vi "snap_usrp_rx.vi"() -> ()   [LabVIEW 2014]
uses:
  <vilib>/vision/Image Controls.llb/IMAQ Image.ctl
  <vilib>/addons/Modulation/Analog/support/mod_Set Error Source.vi
  var_rx_stop.vi
  <vilib>/addons/Modulation/Digital/Support/Common/Validators/mod_Generate Filter Coefficients Validate.vi
  <vilib>/addons/Modulation/Digital/General/subVIs/mod_Generate Filter Coefficients.vi
  <instrlib>/niUSRP/niUSRP Fetch Rx Data (CDB Cluster).vi
  <vilib>/addons/Modulation/niDMT.lvlib
panel:
  out "total_pkts":u32
  in  "arity":enum16{"binary", "quadrature"}(ring)
  out "Image":T1(plugin-control)
  out "# elements in queue":i32
  in  "queue limit":i32
  out "error IO":errorcluster
  in  "number of samples":i64=100000
  in  "Clocking and Synchronization:Timebase Clock Source":string(combo)="Internal"
  in  "Clocking and Synchronization:Reference Frequency Source":string(combo)="Internal"
  in  "Active Channel":string
  in  "active antenna":string
  in  "gain":dbl format="%#_6f"
  in  "carrier frequency":dbl=100000.0 format="%#_6p"
  in  "IQ rate":dbl=100000.0 format="%#_6p"
  in  "device names":refnum<k15>
  in  "stop":bool
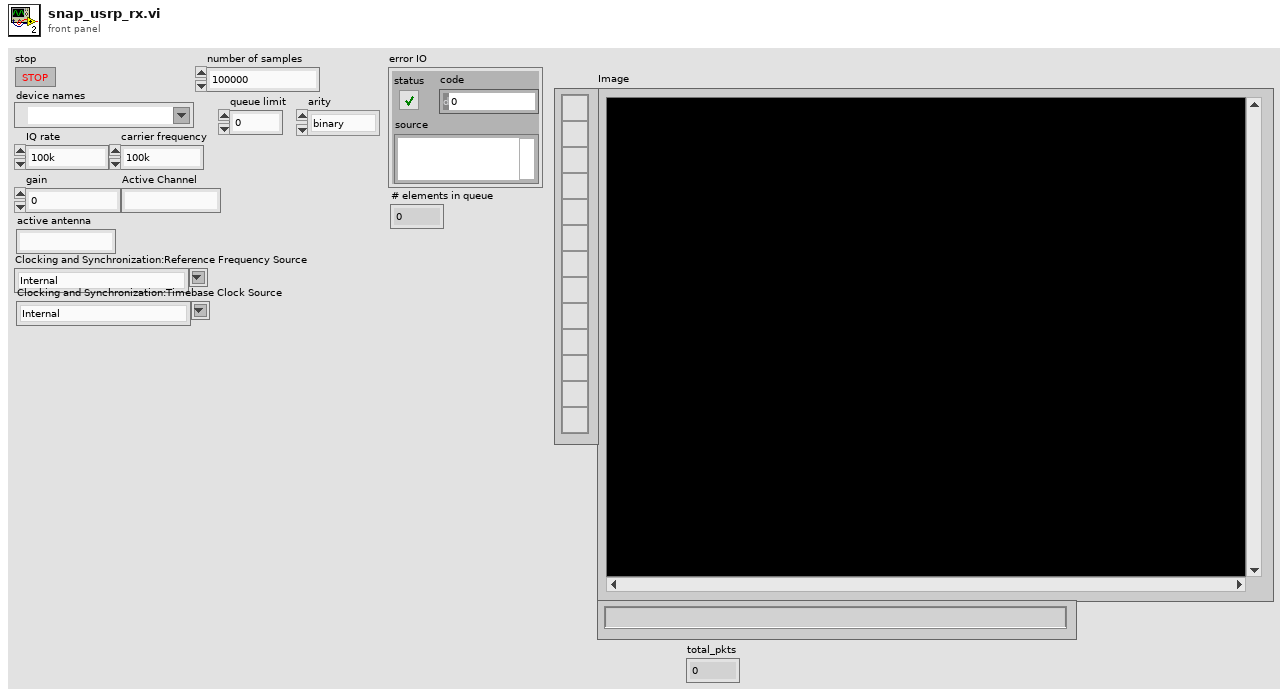
[diagram p1: front panel]
types:
  T1 = typedef "IMAQ Image.ctl" = refnum<image>
  T2 = enum16{"none", "Raised Cosine", "Root Raised Cos", "Gaussian"}
  T3 = enum16{"FSK", "PSK", "QAM", "MSK", "PAM", "ASK", "CPM"}
  T4 = cluster{"pkt_idx":u32, "pkt_size":u32, "payload":string}[]
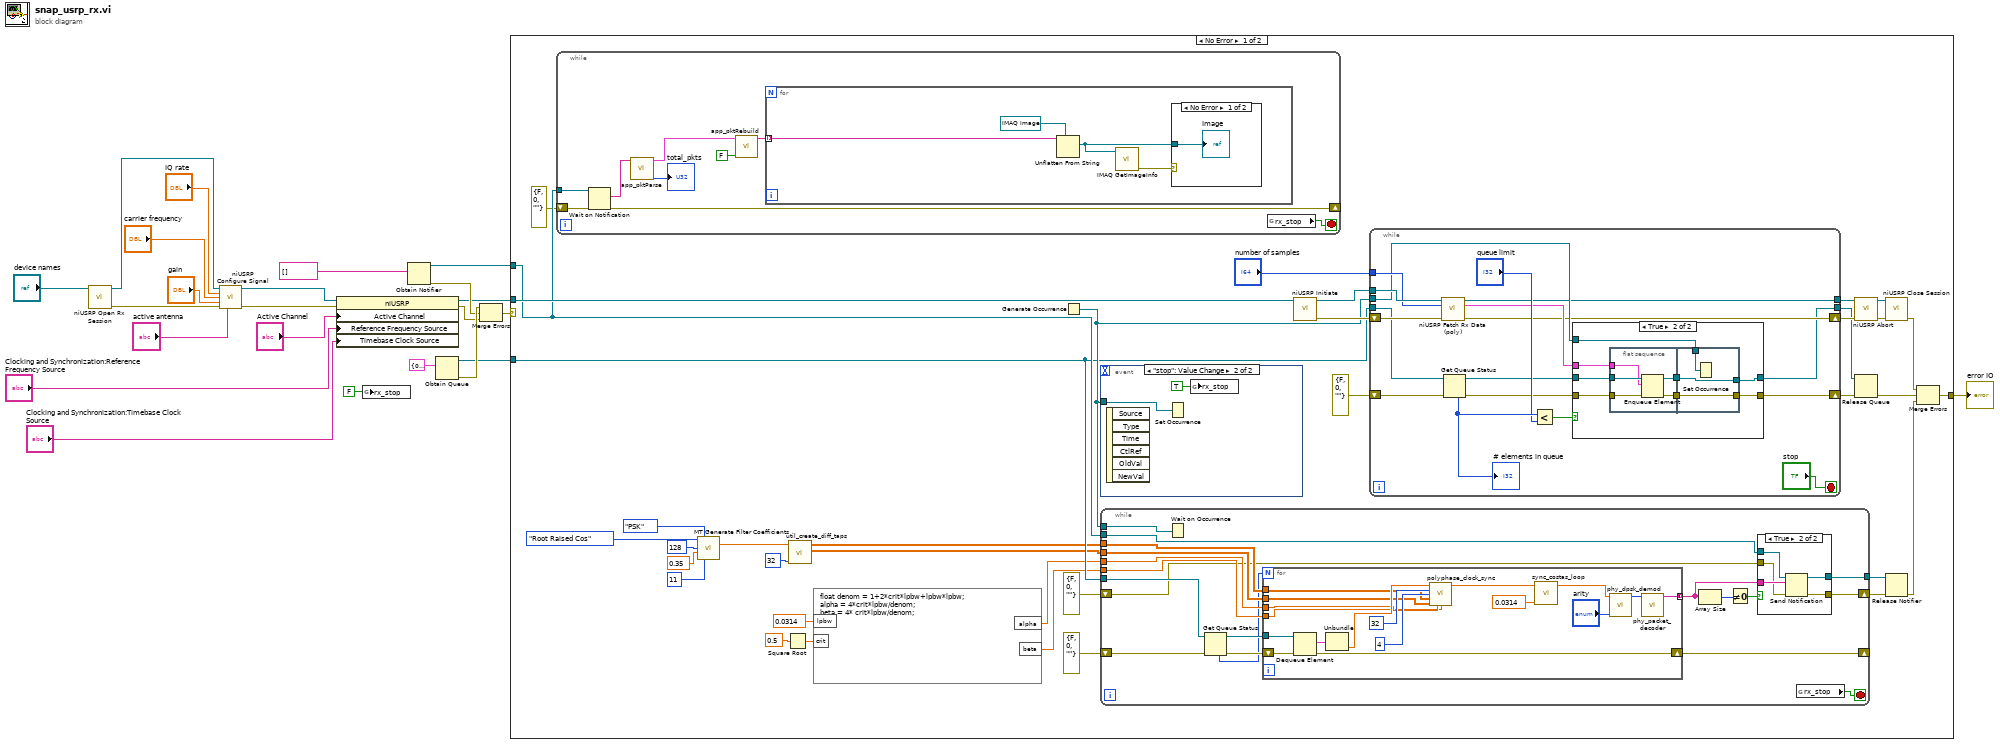
[diagram p0: block diagram]
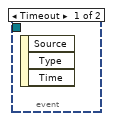
[diagram p5: hidden frame]
diagram:
  n1 = call <instrlib>:"niUSRP Open Rx Session.vi"("device names"="device names") -> ("session handle out"=w22:refnum<k15>, "error out"=w21:errorcluster)  [unwired: 13 in]
  n2 = call <instrlib>:"niUSRP Configure Signal.vi"("session handle"=w22, "IQ rate"="IQ rate", "carrier frequency"="carrier frequency", "gain"="gain", "error in (no error)"=w21, "active antenna"="active antenna") -> ("session handle out"=w20:refnum<k15>, "error out"=w19:errorcluster)  [unwired: 5 in, 3 out]
  n3 = property class="niUSRP"(reference=w20, error in=w19, "Active Channel"="Active Channel", "Reference Frequency Source"="Clocking and Synchronization:Reference Frequency Source", "Timebase Clock Source"="Clocking and Synchronization:Timebase Clock Source") -> (reference out=w6:refnum<k15>, error out=w16:errorcluster)
  n4 = global write "var_rx_stop.vi" "rx_stop"(FALSE) -> ()
  n5 = Obtain Notifier(notification data type=string[] []) -> (notifier out=w3:refnum<notifier>, error out=w17:errorcluster)  [unwired: 3 in, 1 out]
  n6 = Obtain Queue(element data type=cluster{"t0":dbl, "dt":dbl, "Y":cdb[]} {"t0"=0.0, "dt"=0.0, "Y"=[]} ("data")) -> (queue out=w4:refnum<queue>, error out=w18:errorcluster)  [unwired: 4 in, 1 out]
  n7 = Merge Errors(w18, w17, w16) -> (w15:errorcluster)
  n8 = case shown="No Error" w15 {
    selector: w15 -> [_ w155]
    tunnel: w6 -> [w60 _]
    tunnel: w4 -> [w38 _]
    tunnel: w3 -> [w47 _]
    tunnel: [w42 w155] -> w2
    frame No Error {
      n9 = while {
        tunnel: w47 -> [w68]
        shift-right: [w66] -> _
        shift-left: errorcluster {"status"=FALSE, "code"=0, "source"=""} ("error out") -> [w67]
        stop <- w69 stop-if-true
        n10 = Wait on Notification(notifier=w68, error in (no error)=w67) -> (notification=w65:string[], error out=w66:errorcluster)  [unwired: 2 in, 2 out]
        n11 = call "app_pktParse.vi"("pkts_get"=w65) -> ("total_pkts"=→"total_pkts":u32, "app_pkt"=w64:T4)  [unwired: 9 in]
        n12 = call "app_pktRebuild.vi"("reset"=FALSE, "app_pkt"=w64) -> ("out pkts"=w61:string[])  [unwired: 9 in]
        n13 = for {
          tunnel: w61 -> [w73] mode=indexing
          n14 = Unflatten From String(type=T1 refnum ("Image"), binary string=w73) -> (value=w70:T1)  [unwired: 3 in, 2 out]
          n15 = call "IMAQ GetImageInfo"("Image"=w70) -> ("error out"=w71:errorcluster)  [unwired: 3 in, 7 out]
          n16 = case shown="No Error" w71 {
            tunnel: w70 -> [w74 _]
            frame No Error {
              "Image" <- w74
            }
            frame Error {
            }
          }
        }
        n17 = global read "var_rx_stop.vi" "rx_stop"() -> (w69:bool)
      }
      n18 = call <vilib>:"MT Generate Filter Coefficients.vi"("pulse shaping filter (none)"=T2."Root Raised Cos", "modulation type"=T3."PSK", "matched samples per symbol (16)"=128, "filter parameter"=0.35, "filter length (symbols)"=11) -> ("matched filter coefficients"=w33:dbl[])  [unwired: 8 in, 2 out]
      n19 = Square Root(x=0.5) -> (sqrt(x)=w36:dbl)
      n20 = call "util_create_diff_taps.vi"("nfilts"=32, "taps"=w33) -> ("out diff taps"=w24:dbl[][], "out taps"=w25:dbl[][])  [unwired: 7 in, 1 out]
      n21 = formula code="float denom = 1+2*crit*lpbw+lpbw*lpbw;\nalpha = 4*crit*lpbw/denom;\nbeta = 4* crit*lpbw/denom;"("lpbw"=0.0314 ("input variable"), "crit"=w36) -> ("alpha"=w27:dbl, "beta"=w26:dbl)
      n22 = Generate Occurrence() -> (w56:refnum<k4>)
      n23 = event shown="[1] \"stop\": Value Change" {
        selector: _ -> [_ _]
        dyn-events: _ -> [_ _]
        timeout: _ -> [_ _]
        tunnel: w56 -> [_ w153]
        event Timeout {
          n24 = event-data() -> ()  [unwired: 1 in, 3 out]
        }
        event "stop": Value Change {
          n25 = event-data() -> ()  [unwired: 1 in, 6 out]
          n26 = Set Occurrence(w153) -> ()
          n27 = global write "var_rx_stop.vi" "rx_stop"(TRUE) -> ()
        }
      }
      n28 = while {
        tunnel: w56 -> [w93]
        tunnel: w47 -> [w79]
        tunnel: [w76] -> w52
        shift-right: [w77] -> w51
        shift-left: errorcluster {"status"=FALSE, "code"=0, "source"=""} ("error out") -> [w78]
        shift-right: [w83] -> _
        shift-left: errorcluster {"status"=FALSE, "code"=0, "source"=""} ("error out") -> [w91]
        tunnel: w38 -> [w90]
        tunnel: w25 -> [w87]
        tunnel: w24 -> [w86]
        tunnel: w27 -> [w85]
        tunnel: w26 -> [w84]
        stop <- w92 stop-if-true
        n29 = Wait on Occurrence(2:w93) -> ()  [unwired: 2 in, 1 out]
        n30 = Get Queue Status(queue=w90, error in (no error)=w91) -> (queue out=w89:refnum<queue>, error out=w88:errorcluster, # elements in queue=w75:i32)  [unwired: 1 in, 5 out]
        n31 = for {
          N: w75 -> [_]
          tunnel: w89 -> [w117]
          shift-right: [w101] -> w83
          shift-left: w88 -> [w116]
          tunnel: w87 -> [w109]
          tunnel: w86 -> [w108]
          tunnel: w85 -> [w107]
          tunnel: w84 -> [w106]
          tunnel: [w102] -> w82 mode=concatenating
          n32 = Dequeue Element(queue=w117, error in (no error)=w116) -> (element=w115:cluster{"t0":dbl, "dt":dbl, "Y":cdb[]}, error out=w101:errorcluster)  [unwired: 1 in, 2 out]
          n33 = Unbundle(w115) -> ("Y"=w114:cdb[])  [unwired: 2 out]
          n34 = call "polyphase_clock_sync.vi"("samples"=w114, "nfilts"=32, "sps"=4, "taps"=w109, "diff taps"=w108, "alpha"=w107, "beta"=w106) -> ("out symbols"=w113:cdb[])  [unwired: 7 in, 1 out]
          n35 = call "sync_costas_loop.vi"("loop bandwidth"=0.0314, "symbols"=w113) -> ("outputs"=w112:cdb[])  [unwired: 9 in]
          n36 = call "phy_dpsk_demod.vi"("arity"="arity", "dpsk"=w112) -> ("bitstream"=w103:u8[])  [unwired: 9 in]
          n37 = call "phy_packet_decoder.vi"("bits"=w103) -> ("string Array"=w102:string[])  [unwired: 10 in]
        }
        n38 = Array Size(array=w82) -> (size(s)=w81:i32)
        n39 = Not Equal To 0?(x=w81) -> (x != 0?=w80:bool)
        n40 = case shown="True" w80 {
          tunnel: w82 -> [_ w100]
          tunnel: w79 -> [w95 w99]
          tunnel: w78 -> [w94 w98]
          tunnel: [w94 w97] -> w77
          tunnel: [w95 w96] -> w76
          frame False {
          }
          frame True {
            n41 = Send Notification(notification=w100, notifier=w99, error in (no error)=w98) -> (notifier out=w96:refnum<notifier>, error out=w97:errorcluster)
          }
        }
        n42 = global read "var_rx_stop.vi" "rx_stop"() -> (w92:bool)
      }
      n43 = call <instrlib>:"niUSRP Initiate.vi"("session handle"=w60) -> ("session handle out"=w59:refnum<k15>, "error out"=w58:errorcluster)  [unwired: 13 in]
      n44 = while {
        tunnel: w59 -> [w133]
        tunnel: "number of samples" -> [w131]
        tunnel: w56 -> [w130]
        tunnel: w38 -> [w129]
        shift-right: [w121] -> w53
        shift-left: w58 -> [w132]
        shift-right: [w119] -> w40
        shift-left: errorcluster {"status"=FALSE, "code"=0, "source"=""} ("error out") -> [w128]
        tunnel: [w122] -> w41
        tunnel: [w118] -> w39
        stop <- "stop" stop-if-true
        n45 = call-poly <instrlib>:"niUSRP Fetch Rx Data (poly).vi"("session handle"=w133, "number of samples"=w131, "error in (no error)"=w132) -> ("session handle out"=w122:refnum<k15>, "data"=w123:cluster{"t0":dbl, "dt":dbl, "Y":cdb[]}, "error out"=w121:errorcluster)  [unwired: 9 in, 1 out]
        n46 = Get Queue Status(queue=w129, error in (no error)=w128) -> (queue out=w124:refnum<queue>, error out=w120:errorcluster, # elements in queue=w127:i32)  [unwired: 1 in, 5 out]
        "# elements in queue" <- w127
        n47 = Less?(x=w127, y="queue limit") -> (x < y?=w125:bool)
        n48 = case shown="True" w125 {
          tunnel: w130 -> [_ w137]
          tunnel: w124 -> [w135 w144]
          tunnel: w123 -> [_ w143]
          tunnel: w120 -> [w136 w142]
          tunnel: [w136 w141] -> w119
          tunnel: [w135 w140] -> w118
          frame False {
          }
          frame True {
            n49 = flat-sequence {
              tunnel: w144 -> [w149]
              tunnel: w143 -> [w148]
              tunnel: w142 -> [w147]
              tunnel: [w146] -> w139
              tunnel: [w145] -> w138
              tunnel: [w151] -> w140
              tunnel: [w152] -> w141
              tunnel: w139 -> [w152]
              tunnel: w138 -> [w151]
              tunnel: w137 -> [w150]
              frame #0 {
                n50 = Enqueue Element(queue=w149, element=w148, error in (no error)=w147) -> (queue out=w145:refnum<queue>, error out=w146:errorcluster)  [unwired: 1 in, 1 out]
              }
              frame #1 {
                n51 = Set Occurrence(w150) -> ()
              }
            }
          }
        }
      }
      n52 = call <instrlib>:"niUSRP Abort.vi"("session handle"=w41, "error in (no error)"=w53) -> ("session handle out"=w55:refnum<k15>, "error out"=w54:errorcluster)  [unwired: 12 in]
      n53 = Release Queue(queue=w39, error in (no error)=w40) -> (error out=w49:errorcluster)  [unwired: 1 in, 2 out]
      n54 = call <instrlib>:"niUSRP Close Session.vi"("session handle"=w55, "error in (no error)"=w54) -> ("error out"=w50:errorcluster)  [unwired: 13 in]
      n55 = Release Notifier(notifier=w52, error in (no error)=w51) -> (error out=w48:errorcluster)  [unwired: 1 in, 2 out]
      n56 = Merge Errors(w50, w49, w48) -> (w42:errorcluster)
    }
    frame Error {
    }
  }
  "error IO" <- w2
